vi "demo_Community Training Initiative (CTI).vi"(11 "Stop Demo":refnum<user-event>) -> ()   [LabVIEW 2020]
panel:
  # "Make LabVIEW available to Anyone, Anywhere at the lowest price-point ever. \n\nIt is currently concentrating on open-source training materials and low-cost training platforms, hopefully removing the cost of entry to the world of graphical programming.\n\nIt currently consists of a website for the course materials (here), a downloadable virtual machine image with LabVIEW for Linux loaded (kindly hosted by GCentral) and firmware to convert a Raspberry Pi Pico into a SCPI VISA Instrument."
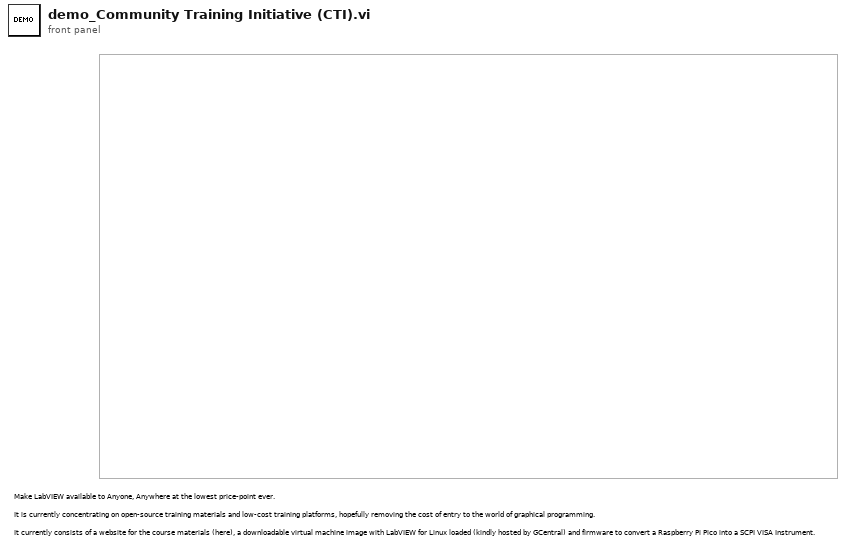
[diagram p1: front panel]
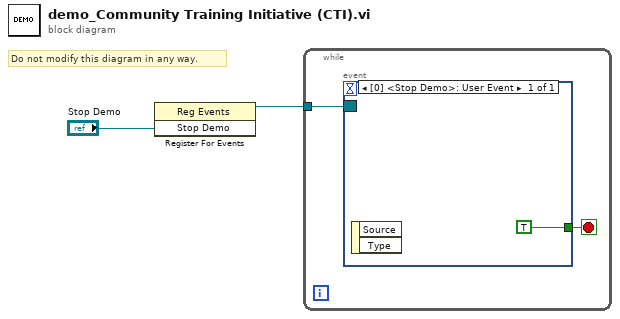
[diagram p0: block diagram]
diagram:
  # "Do not modify this diagram in any way."
  n1 = register-events("Stop Demo") -> (reference out=w1:refnum<event-registration>)  [unwired: 2 in, 1 out]
  n2 = while {
    tunnel: w1 -> [w4]
    stop <- w3 stop-if-true
    n3 = event shown="[0] <Stop Demo>: User Event" {
      selector: w4 -> [_]
      dyn-events: _ -> [_]
      timeout: _ -> [_]
      tunnel: [TRUE] -> w3
      event User Event {
        n4 = event-data() -> ()  [unwired: 1 in, 2 out]
      }
    }
  }
